vi "sample0(Basic).vi"   [LabVIEW 2011]
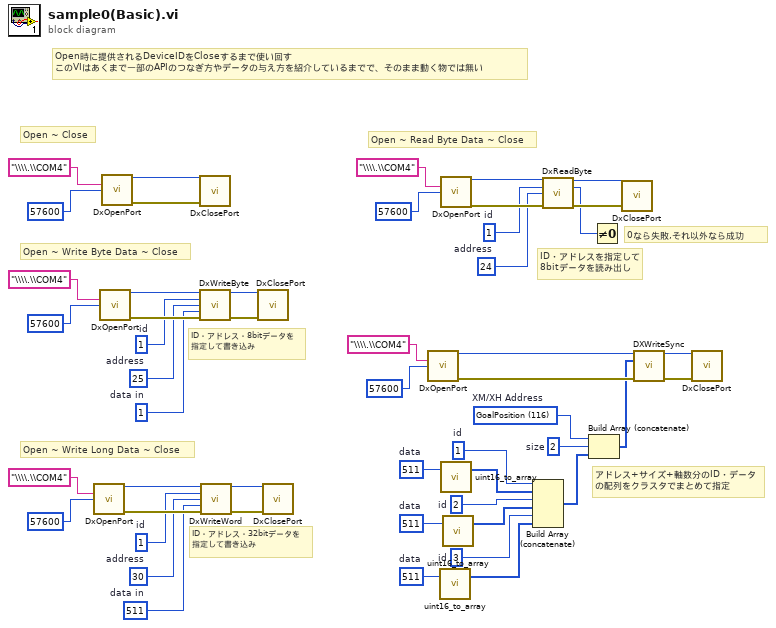
[diagram p0: block diagram]
diagram:
  w6 = u8 1  # id
  w2 = u8 3  # id
  w4 = u8 2  # id
  w11 = u16 511  # data
  w12 = u16 511  # data
  w50 = u16 511  # data
  w7 = u8 116 items=["ModelNo"=0, "ModelInfo"=2, "VersionOfFirmware"=6, "ID"=7, "Baudrate"=8, "ReturnDelayTime"=9, "OperationMode"=11, "ProtocolVersion"=13, "HormingOffset"=20, "MovingThreshold"=24, "TemperatureLimit"=31, "MaxVoltageLimit"=32, "MinVoltageLimit"=34, "PWMLimit"=36, "CurrentLimit"=38, "AccelerationLimit"=40, "VelocityLimit"=44, "MaxPositionLimit"=48, "MinPositionLimit"=52, "Shutdown"=63, "TorqueEnable"=64, "LED"=65, "StatusReturnLevel"=68, "RegistedInstruction"=69, "HardwareErrorStatus"=70, "VelocityIGain"=76, "VelocityPGain"=78, "VelocityDGain"=80, "PositionIGain"=82, "PositionPGain"=84, "FeedForward2ndGain"=88, "FeedForward1stGain"=90, "GoalPWM"=100, "GoalCurrent"=102, "GoalVelocity"=104, "ProfileAcceleration"=108, "ProfileVelocity"=112, "GoalPosition"=116, "RealtimeTick"=120, "Moving"=122, "MovingStatus"=123, "PresentPWM"=124, "PresentCurrent"=126, "Presentvelocity"=128, "PresentPosition"=132, "VelocityTrajectory"=136, "PositionTrajectory"=140, "PresentIInputVoltage"=144, "PresentTemperature"=146]  # XM/XH Address
  w8 = u8 2  # size
  w13 = u16 24  # address
  w14 = u8 1  # id
  w15 = u16 511  # data in
  w16 = u16 30  # address
  w17 = u8 1  # id
  w18 = u8 1  # data in
  w19 = u16 25  # address
  w20 = u8 1  # id
  # "0なら失敗,それ以外なら成功"
  # "ID・アドレスを指定して\n8bitデータを読み出し"
  # "ID・アドレス・8bitデータを\n指定して書き込み"
  # "ID・アドレス・32bitデータを\n指定して書き込み"
  # "アドレス+サイズ+軸数分のID・データ\nの配列をクラスタでまとめて指定"
  # "Open ~ Read Byte Data ~ Close"
  # "Open ~ Write Long Data ~ Close"
  # "Open ~ Write Byte Data ~ Close"
  # "Open ~ Close"
  # "Open時に提供されるDeviceIDをCloseするまで使い回す\nこのVIはあくまで一部のAPIのつなぎ方やデータの与え方を紹介しているまでで、そのまま動く物では無い"
  n1 = call "DxOpenPort.vi"("port"="\\\\.\\COM4", "baudrate"=u32 57600) -> ("dvid"=w33:u32, "エラー出力"=w31:errorcluster)  [unwired: 11 in, 1 out]
  n2 = call "DxOpenPort.vi"("port"="\\\\.\\COM4", "baudrate"=u32 57600) -> ("dvid"=w37:u32, "エラー出力"=w35:errorcluster)  [unwired: 11 in, 1 out]
  n3 = call "DxOpenPort.vi"("port"="\\\\.\\COM4", "baudrate"=u32 57600) -> ("dvid"=w39:u32, "エラー出力"=w38:errorcluster)  [unwired: 11 in, 1 out]
  n4 = call "DxClosePort.vi"("dvid"=w39, "エラー入力"=w38) -> ()  [unwired: 12 in, 2 out]
  n5 = call "DxWriteByte.vi"("dvid in"=w37, "id"=w20, "address"=w19, "data in"=w18, "エラー入力"=w35) -> ("dvid out"=w36:u32, "エラー出力"=w34:errorcluster)  [unwired: 8 in, 1 out]
  n6 = call "DxWriteWord.vi"("dvid in"=w33, "id"=w17, "address"=w16, "data in"=w15, "エラー入力"=w31) -> ("dvid out"=w32:u32, "エラー出力"=w30:errorcluster)  [unwired: 8 in, 1 out]
  n7 = call "DxClosePort.vi"("dvid"=w36, "エラー入力"=w34) -> ()  [unwired: 12 in, 2 out]
  n8 = call "DxClosePort.vi"("dvid"=w32, "エラー入力"=w30) -> ()  [unwired: 12 in, 2 out]
  n9 = call "DxOpenPort.vi"("port"="\\\\.\\COM4", "baudrate"=u32 57600) -> ("dvid"=w29:u32, "エラー出力"=w27:errorcluster)  [unwired: 11 in, 1 out]
  n10 = call "uint16_to_array.vi"("uint16"=w11) -> ("array"=w1:u8[])  [unwired: 2 in]
  n11 = call "DxOpenPort.vi"("port"="\\\\.\\COM4", "baudrate"=u32 57600) -> ("dvid"=w25:u32, "エラー出力"=w22:errorcluster)  [unwired: 11 in, 1 out]
  n12 = call "uint16_to_array.vi"("uint16"=w50) -> ("array"=w5:u8[])  [unwired: 2 in]
  n13 = call "uint16_to_array.vi"("uint16"=w12) -> ("array"=w3:u8[])  [unwired: 2 in]
  n14 = Build Array (concatenate)(w6, w5, w4, w3, w2, w1) -> (w10:u8[])
  n15 = call "DxReadByte.vi"("dvid in"=w25, "id"=w14, "address"=w13, "エラー入力"=w22) -> ("dvid out"=w24:u32, "data out"=w21:u8, "エラー出力"=w23:errorcluster)  [unwired: 8 in, 1 out]
  n16 = Build Array (concatenate)(w7, w8, w10) -> (w9:u8[])
  n17 = Not Equal To 0?(x=w21) -> ()  [unwired: 1 out]
  n18 = call "DxClosePort.vi"("dvid"=w24, "エラー入力"=w23) -> ()  [unwired: 12 in, 2 out]
  n19 = call "DXWriteSync.vi"("dvid in"=w29, "data in"=w9, "エラー入力"=w27) -> ("dvid out"=w28:u32, "エラー出力"=w26:errorcluster)  [unwired: 10 in, 1 out]
  n20 = call "DxClosePort.vi"("dvid"=w28, "エラー入力"=w26) -> ()  [unwired: 12 in, 2 out]
